vi "SetParam.vi"(8 "error in (no error)":errorcluster caption="entrée d'erreur (pas d'erreur)", 10 "make_biclusters":T1={"n_rows"=300, "n_cols"=300, "n_clusters"=5, "noise"=5.0, "minval"=10, "maxval"=100, "shuffle"=TRUE, "random_state"=-1, "Returns"="X"} {"random_state" min=-1; "n_clusters" min=1; "n_cols" min=1; "n_rows" min=1}, 11 "Biclusters.lvclass":refnum<class "Biclusters.lvclass">) -> (0 "error out":errorcluster caption="sortie d'erreur", 3 "Biclusters.lvclass":refnum<class "Biclusters.lvclass">)   [LabVIEW 2020, in "Biclusters.lvclass"]
doc: "Set Parameters"
uses:
  Biclusters.lvclass
  Biclusters.lvclass/Biclusters.ctl
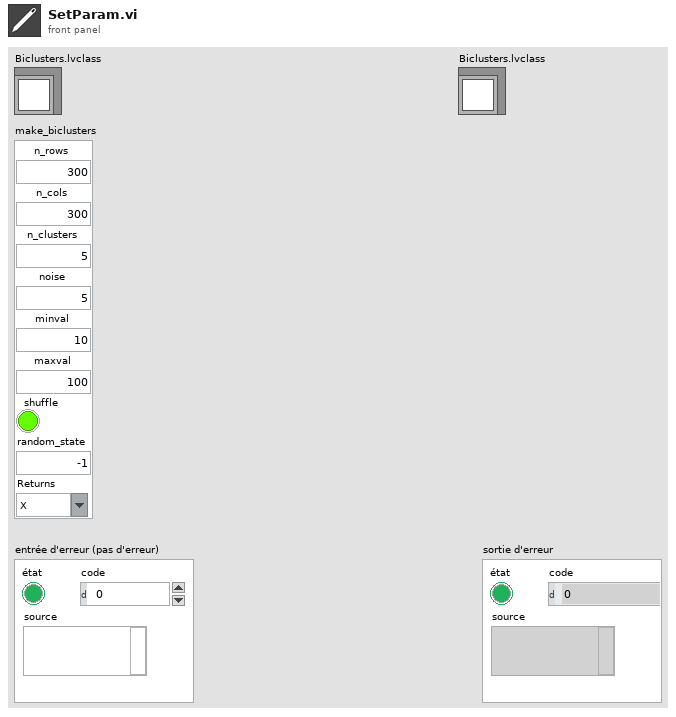
[diagram p1: front panel]
types:
  T1 = cluster{"n_rows":u32, "n_cols":u32, "n_clusters":u32, "noise":dbl, "minval":i32, "maxval":i32, "shuffle":bool, "random_state":i32, "Returns":string}
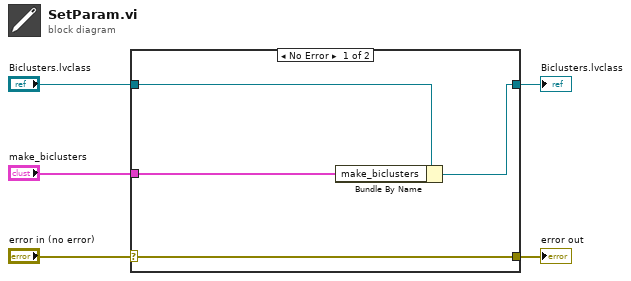
[diagram p0: block diagram]
diagram:
  n1 = case shown="No Error" "error in (no error)" {
    selector: "error in (no error)" -> [w9 w10]
    tunnel: [w9 w10] -> w4
    tunnel: [w7 w11] -> w2
    tunnel: "Biclusters.lvclass" -> [w8 w11]
    tunnel: "make_biclusters" -> [w6 _]
    frame No Error {
      n2 = Bundle By Name(cluster=w8, "make_biclusters"=w6) -> (w7:refnum<class "Biclusters.lvclass">)
    }
    frame Error {
    }
  }
  "error out" <- w4
  "Biclusters.lvclass" <- w2
